vi "E725_All_VIs.vi"   [LabVIEW 2015]
doc: "This VI contains all high level and low level VIs valid for E-725. \nSee diagram for a survey of all E-725 high level and low level VIs. \nMenu / Browse / Show VI Hierarchy will show the file paths of the VIs. \nGlobal Variables are shown as Control as well as Indicator."
uses:
  Low Level/General command.llb/Controller names.ctl
  Low Level/Communication.llb/Available DLL interfaces.ctl
  Low Level/Communication.llb/Available DLLs.ctl
  Low Level/Communication.llb/Available interfaces.ctl
  Low Level/Communication.llb/Termination character.ctl
  Low Level/Analog control.llb/Available Analog Commands.ctl
  Low Level/Communication.llb/Global1.vi
  Low Level/General command.llb/Global2 (Array).vi
  Low Level/Communication.llb/Global DaisyChain.vi
  Low Level/Analog control.llb/Global Analog.vi
  Low Level/Support.llb/Unbunde/bundle interface clusters for PI Terminal.vi
panel:
  # "E-725 PI GCS LabVIEW driver set"
  # "This VI contains all high level and low level VIs valid for E-725. See diagram for a survey\nof all E-725 high level and low level VIs. Menu / Browse / Show VI Hierarchy will show\nthe file paths of the VIs. Global Variables are shown as Control as well as Indicator."
types:
  T1 = typedef "Available Analog Commands.ctl" = enum16{"INITIALIZE", "VOL?", "VOL ", "CLOSE", "MOV", "POS?", "VCO", "VCO?", "WAIT_WF", "TMN?", "TMX?", "VEL", "VEL?", "SAI?", "MVR", "ERR?", "#24", "STP", "*IDN?", "#5", "STE", "DRR?", "W_Wave", "HLP?", "W/R_Wave"}
  T2 = typedef "Termination character.ctl" = enum16{"LF", "CR", "LFCR", "CRLF"}
  T3 = typedef "Available interfaces.ctl" = u16
  T4 = typedef "Available DLLs.ctl" = u16
  T5 = typedef "Available DLL interfaces.ctl" = u16
  T6 = typedef "Controller names.ctl" = enum16{"None", "Analog", "C-702", "C-843", "C-843.PM", "C-844", "C-848", "C-865", "C-866", "C-867", "C-880", "E-516", "E-517", "E-710", "E-712", "E-725", "E-753", "E-755", "E-761", "E-816", "E-861", "F-206", "M-840", "M-850", "M-8X0", "Mercury"}
  T7 = cluster{"Conversion factor":dbl[], "Velocity":dbl[], "Velocity control mode":bool, "AO.Resolution":dbl, "Lower voltage limit (V)":dbl, "Upper voltage limit (V)":dbl, "AO_WF_T (s)":dbl, "AI Sample Rate":dbl, "AI Samples/Channel":i32, "Hyperbit":bool, "Offset (V)":dbl[], "Hyperbit StayOnPos":bool, "Gain (V)":dbl[], "Bit rate (Hz)":dbl, "PWM rate (Hz)":dbl, "HyperBit Password":string, "AO.MaxRate":dbl, "Conversion offset":dbl[]}[]
  T8 = cluster{"No. of devices":i32, "Port ID":i32, "Devices":string[], "Description":string}[]
  T9 = cluster{"Conn. axes":string[], "Controller name":T6}[]
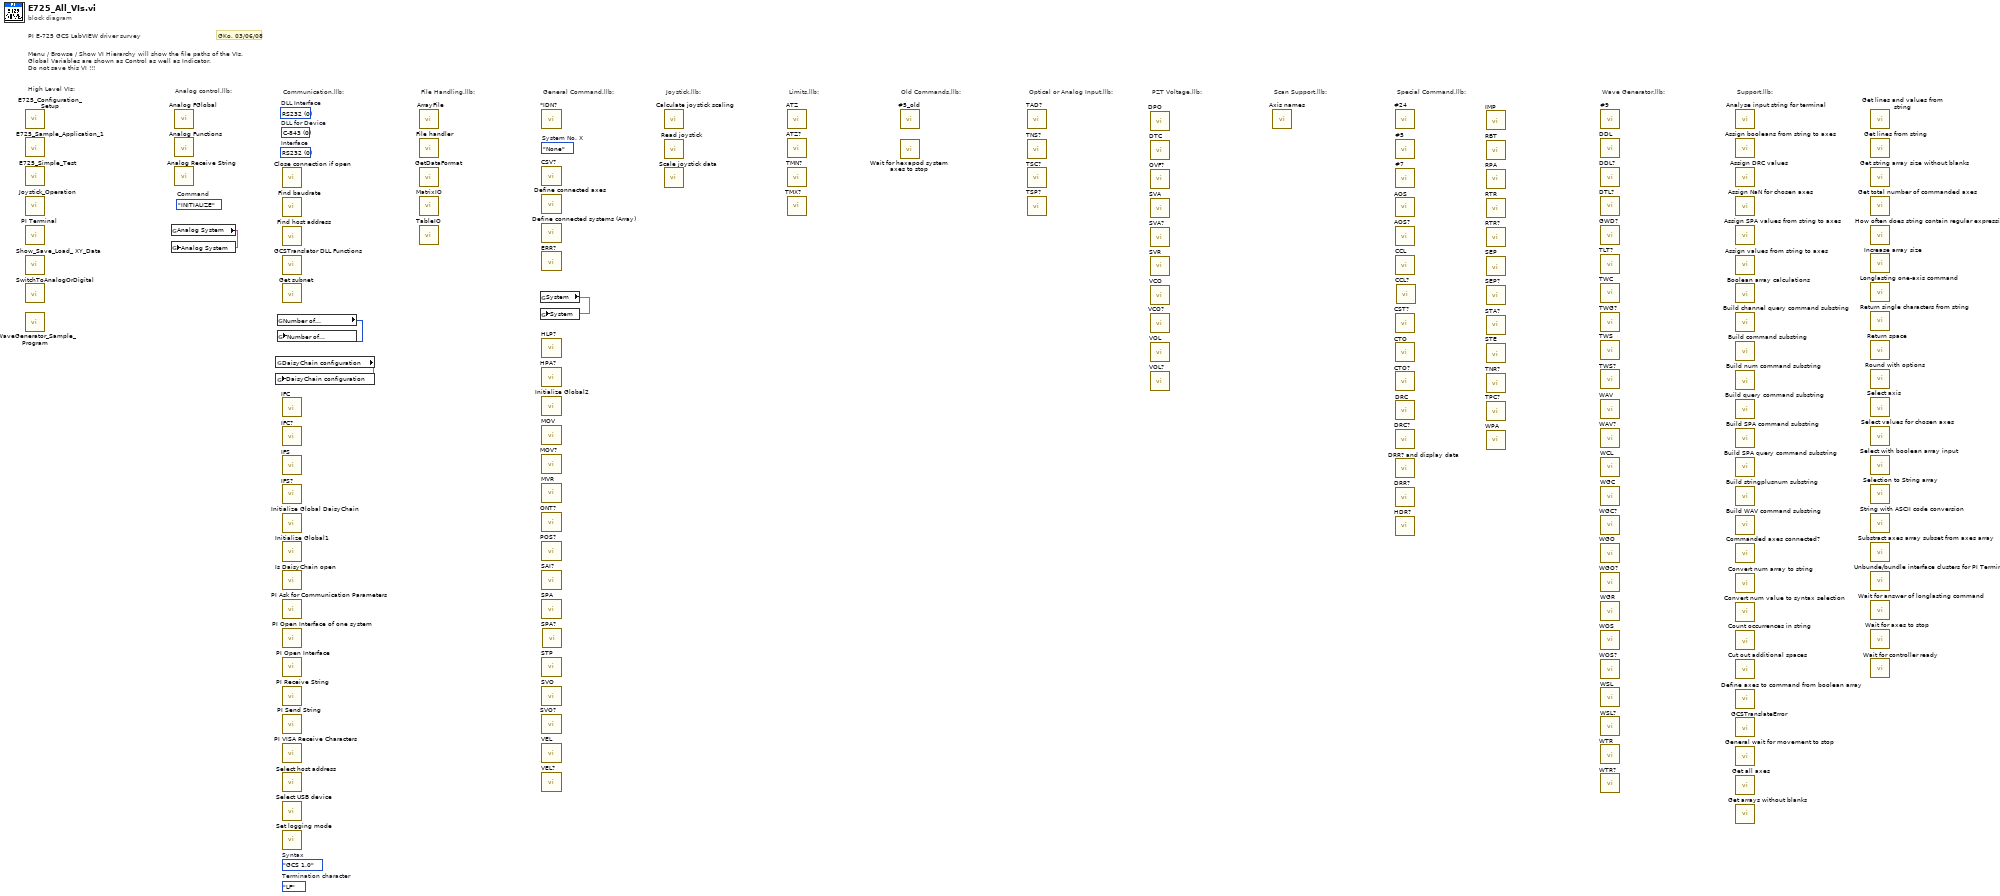
[diagram p0: block diagram]
diagram:
  (unwired) enum16{"GCS 1.0", "GCS 2.0"}."GCS 1.0"  # Syntax
  (unwired) Available_Analog_Commands."INITIALIZE"  # Command
  (unwired) Termination_character."LF"  # Termination character
  (unwired) T3 0 items=["RS232", "GPIB", "DLL", "TCP-IP"]  # Interface
  (unwired) T4 0 items=["C-843", "C-844", "E-710", "C-843.PM", "C-865", "E-761", "Mercury", "E-755", "E-753", "C-866", "E-712", "E-725", "E-861", "C-867", "E-517"]  # DLL for Device
  (unwired) T5 0 items=["RS232", "GPIB", "Board", "TCP-IP", "USB"]  # DLL Interface
  (unwired) Controller_names."None"  # System No. X
  # "GKo, 03/06/08"
  # "High Level VIs:"
  # "Analog control.llb:"
  # "Wave Generator.llb:"
  # "Support.llb:"
  # "Special Command.llb:"
  # "Scan Support.llb:"
  # "PZT Voltage.llb:"
  # "Optical or Analog Input.llb:"
  # "Old Commands.llb:"
  # "Limits.llb:"
  # "Joystick.llb:"
  # "General Command.llb:"
  # "File Handling.llb:"
  # "Menu / Browse / Show VI Hierarchy will show the file paths of the VIs. \nGlobal Variables are shown as Control as well as Indicator.\nDo not save this VI !!!"
  # "PI E-725 GCS LabVIEW driver survey"
  # "Communication.llb:"
  n1 = call "E725_Configuration_Setup.vi"() -> ()  [unwired: 15 in, 5 out]
  n2 = call "E725_Sample_Application_1.vi"() -> ()  [unwired: 1 in]
  n3 = call "E725_Simple_Test.vi"() -> ()  [unwired: 15 in, 5 out]
  n4 = call "Joystick_Operation.vi"() -> ()  [unwired: 19 in, 1 out]
  n5 = call "PI Terminal.vi"() -> ()  [unwired: 20 in]
  n6 = call "Show_Save_Load_ XY_Data.vi"() -> ()  [unwired: 19 in, 1 out]
  n7 = call "SwitchToAnalogOrDigital.vi"() -> ()  [unwired: 17 in, 3 out]
  n8 = call "WaveGenerator_Sample_Program.vi"() -> ()  [unwired: 18 in, 2 out]
  n9 = global read "Global Analog.vi" "Analog System"() -> (w1:T7)
  n10 = global write "Global Analog.vi" "Analog System"(w1) -> ()
  n11 = call "Analog FGlobal.vi"() -> ()  [unwired: 19 in, 1 out]
  n12 = call "Analog Functions.vi"() -> ()  [unwired: 17 in, 3 out]
  n13 = call "Analog Receive String.vi"() -> ()  [unwired: 18 in, 2 out]
  n14 = global read "Global DaisyChain.vi" "DaisyChain configuration"() -> (w2:T8)
  n15 = global write "Global DaisyChain.vi" "DaisyChain configuration"(w2) -> ()
  n16 = global read "Global1.vi" "Number of\nsystems"() -> (w4:i32)
  n17 = global write "Global1.vi" "Number of\nsystems"(w4) -> ()
  n18 = call "Close connection if open.vi"() -> ()  [unwired: 18 in, 2 out]
  n19 = call "Find baudrate.vi"() -> ()  [unwired: 17 in, 3 out]
  n20 = call "Find host address.vi"() -> ()  [unwired: 15 in, 5 out]
  n21 = call "GCSTranslator DLL Functions.vi"() -> ()  [unwired: 15 in, 5 out]
  n22 = call "Get subnet.vi"() -> ()  [unwired: 19 in, 1 out]
  n23 = call "IFC.vi"() -> ()  [unwired: 19 in, 1 out]
  n24 = call "IFC?.vi"() -> ()  [unwired: 18 in, 2 out]
  n25 = call "IFS.vi"() -> ()  [unwired: 19 in, 1 out]
  n26 = call "IFS?.vi"() -> ()  [unwired: 18 in, 2 out]
  n27 = call "Initialize Global DaisyChain.vi"() -> ()  [unwired: 19 in, 1 out]
  n28 = call "Initialize Global1.vi"() -> ()  [unwired: 19 in, 1 out]
  n29 = call "Is DaisyChain open.vi"() -> ()  [unwired: 17 in, 3 out]
  n30 = call "PI Ask for Communication Parameters.vi"() -> ()  [unwired: 12 in, 8 out]
  n31 = call "PI Open Interface of one system.vi"() -> ()  [unwired: 18 in, 2 out]
  n32 = call "PI Open Interface.vi"() -> ()  [unwired: 18 in, 2 out]
  n33 = call "PI Receive String.vi"() -> ()  [unwired: 17 in, 3 out]
  n34 = call "PI Send String.vi"() -> ()  [unwired: 19 in, 1 out]
  n35 = call "PI VISA Receive Characters.vi"() -> ()  [unwired: 17 in, 3 out]
  n36 = call "Select host address.vi"() -> ()  [unwired: 17 in, 3 out]
  n37 = call "Select USB device.vi"() -> ()  [unwired: 17 in, 3 out]
  n38 = call "Set logging mode.vi"() -> ()  [unwired: 19 in, 1 out]
  n39 = call "ArrayFile.vi"() -> ()  [unwired: 18 in, 2 out]
  n40 = call "File handler.vi"() -> ()  [unwired: 17 in, 3 out]
  n41 = call "GetDataFormat.vi"() -> ()  [unwired: 12 in, 8 out]
  n42 = call "MatrixIO.vi"() -> ()  [unwired: 13 in, 7 out]
  n43 = call "TableIO.vi"() -> ()  [unwired: 14 in, 6 out]
  n44 = global read "Global2 (Array).vi" "System"() -> (w3:T9)
  n45 = global write "Global2 (Array).vi" "System"(w3) -> ()
  n46 = call "*IDN?.vi"() -> ()  [unwired: 18 in, 2 out]
  n47 = call "CSV?.vi"() -> ()  [unwired: 18 in, 2 out]
  n48 = call "Define connected axes.vi"() -> ()  [unwired: 18 in, 2 out]
  n49 = call "Define connected systems (Array).vi"() -> ()  [unwired: 19 in, 1 out]
  n50 = call "ERR?.vi"() -> ()  [unwired: 18 in, 2 out]
  n51 = call "HLP?.vi"() -> ()  [unwired: 18 in, 2 out]
  n52 = call "HPA?.vi"() -> ()  [unwired: 18 in, 2 out]
  n53 = call "Initialize Global2.vi"() -> ()  [unwired: 19 in, 1 out]
  n54 = call "MOV.vi"() -> ()  [unwired: 19 in, 1 out]
  n55 = call "MOV?.vi"() -> ()  [unwired: 18 in, 2 out]
  n56 = call "MVR.vi"() -> ()  [unwired: 19 in, 1 out]
  n57 = call "ONT?.vi"() -> ()  [unwired: 18 in, 2 out]
  n58 = call "POS?.vi"() -> ()  [unwired: 18 in, 2 out]
  n59 = call "SAI?.vi"() -> ()  [unwired: 18 in, 2 out]
  n60 = call "SPA.vi"() -> ()  [unwired: 18 in, 2 out]
  n61 = call "STP.vi"() -> ()  [unwired: 19 in, 1 out]
  n62 = call "SVO.vi"() -> ()  [unwired: 19 in, 1 out]
  n63 = call "SVO?.vi"() -> ()  [unwired: 18 in, 2 out]
  n64 = call "VEL.vi"() -> ()  [unwired: 18 in, 2 out]
  n65 = call "VEL?.vi"() -> ()  [unwired: 18 in, 2 out]
  n66 = call "SPA?.vi"() -> ()  [unwired: 14 in, 6 out]
  n67 = call "Calculate joystick scaling.vi"() -> ()  [unwired: 10 in, 10 out]
  n68 = call "Read joystick.vi"() -> ()  [unwired: 15 in, 5 out]
  n69 = call "Scale joystick data.vi"() -> ()  [unwired: 18 in, 2 out]
  n70 = call "ATZ.vi"() -> ()  [unwired: 18 in, 2 out]
  n71 = call "ATZ?.vi"() -> ()  [unwired: 18 in, 2 out]
  n72 = call "TMN?.vi"() -> ()  [unwired: 18 in, 2 out]
  n73 = call "TMX?.vi"() -> ()  [unwired: 18 in, 2 out]
  n74 = call "#5_old.vi"() -> ()  [unwired: 16 in, 4 out]
  n75 = call "Wait for hexapod system axes to stop.vi"() -> ()  [unwired: 18 in, 2 out]
  n76 = call "TAD?.vi"() -> ()  [unwired: 18 in, 2 out]
  n77 = call "TNS?.vi"() -> ()  [unwired: 18 in, 2 out]
  n78 = call "TSC?.vi"() -> ()  [unwired: 18 in, 2 out]
  n79 = call "TSP?.vi"() -> ()  [unwired: 18 in, 2 out]
  n80 = call "DPO.vi"() -> ()  [unwired: 19 in, 1 out]
  n81 = call "DTC.vi"() -> ()  [unwired: 19 in, 1 out]
  n82 = call "OVF?.vi"() -> ()  [unwired: 18 in, 2 out]
  n83 = call "SVA.vi"() -> ()  [unwired: 19 in, 1 out]
  n84 = call "SVA?.vi"() -> ()  [unwired: 18 in, 2 out]
  n85 = call "SVR.vi"() -> ()  [unwired: 19 in, 1 out]
  n86 = call "VCO.vi"() -> ()  [unwired: 19 in, 1 out]
  n87 = call "VCO?.vi"() -> ()  [unwired: 18 in, 2 out]
  n88 = call "VOL.vi"() -> ()  [unwired: 19 in, 1 out]
  n89 = call "VOL?.vi"() -> ()  [unwired: 18 in, 2 out]
  n90 = call "Axis names.vi"() -> ()  [unwired: 17 in, 3 out]
  n91 = call "#24.vi"() -> ()  [unwired: 19 in, 1 out]
  n92 = call "#5.vi"() -> ()  [unwired: 18 in, 2 out]
  n93 = call "#7.vi"() -> ()  [unwired: 17 in, 3 out]
  n94 = call "AOS.vi"() -> ()  [unwired: 19 in, 1 out]
  n95 = call "AOS?.vi"() -> ()  [unwired: 18 in, 2 out]
  n96 = call "CCL.vi"() -> ()  [unwired: 18 in, 2 out]
  n97 = call "CST?.vi"() -> ()  [unwired: 18 in, 2 out]
  n98 = call "CTO.vi"() -> ()  [unwired: 18 in, 2 out]
  n99 = call "CTO?.vi"() -> ()  [unwired: 18 in, 2 out]
  n100 = call "DRC.vi"() -> ()  [unwired: 18 in, 2 out]
  n101 = call "DRC?.vi"() -> ()  [unwired: 16 in, 4 out]
  n102 = call "DRR? and display data.vi"() -> ()  [unwired: 16 in, 4 out]
  n103 = call "DRR?.vi"() -> ()  [unwired: 16 in, 4 out]
  n104 = call "HDR?.vi"() -> ()  [unwired: 18 in, 2 out]
  n105 = call "CCL?.vi"() -> ()  [unwired: 18 in, 2 out]
  n106 = call "IMP.vi"() -> ()  [unwired: 19 in, 1 out]
  n107 = call "RBT.vi"() -> ()  [unwired: 19 in, 1 out]
  n108 = call "RPA.vi"() -> ()  [unwired: 18 in, 2 out]
  n109 = call "RTR.vi"() -> ()  [unwired: 18 in, 2 out]
  n110 = call "RTR?.vi"() -> ()  [unwired: 18 in, 2 out]
  n111 = call "SEP.vi"() -> ()  [unwired: 18 in, 2 out]
  n112 = call "SEP?.vi"() -> ()  [unwired: 14 in, 6 out]
  n113 = call "STA?.vi"() -> ()  [unwired: 18 in, 2 out]
  n114 = call "STE.vi"() -> ()  [unwired: 19 in, 1 out]
  n115 = call "TNR?.vi"() -> ()  [unwired: 18 in, 2 out]
  n116 = call "TPC?.vi"() -> ()  [unwired: 18 in, 2 out]
  n117 = call "WPA.vi"() -> ()  [unwired: 18 in, 2 out]
  n118 = call "#9.vi"() -> ()  [unwired: 18 in, 2 out]
  n119 = call "DDL.vi"() -> ()  [unwired: 19 in, 1 out]
  n120 = call "DDL?.vi"() -> ()  [unwired: 18 in, 2 out]
  n121 = call "DTL?.vi"() -> ()  [unwired: 18 in, 2 out]
  n122 = call "GWD?.vi"() -> ()  [unwired: 18 in, 2 out]
  n123 = call "TLT?.vi"() -> ()  [unwired: 18 in, 2 out]
  n124 = call "TWC.vi"() -> ()  [unwired: 19 in, 1 out]
  n125 = call "TWG?.vi"() -> ()  [unwired: 18 in, 2 out]
  n126 = call "TWS.vi"() -> ()  [unwired: 18 in, 2 out]
  n127 = call "TWS?.vi"() -> ()  [unwired: 18 in, 2 out]
  n128 = call "WAV.vi"() -> ()  [unwired: 26 in, 2 out]
  n129 = call "WAV?.vi"() -> ()  [unwired: 18 in, 2 out]
  n130 = call "WCL.vi"() -> ()  [unwired: 19 in, 1 out]
  n131 = call "WGC.vi"() -> ()  [unwired: 18 in, 2 out]
  n132 = call "WGC?.vi"() -> ()  [unwired: 18 in, 2 out]
  n133 = call "WGO.vi"() -> ()  [unwired: 18 in, 2 out]
  n134 = call "WGO?.vi"() -> ()  [unwired: 18 in, 2 out]
  n135 = call "WGR.vi"() -> ()  [unwired: 19 in, 1 out]
  n136 = call "WOS.vi"() -> ()  [unwired: 19 in, 1 out]
  n137 = call "WOS?.vi"() -> ()  [unwired: 18 in, 2 out]
  n138 = call "WSL.vi"() -> ()  [unwired: 19 in, 1 out]
  n139 = call "WSL?.vi"() -> ()  [unwired: 18 in, 2 out]
  n140 = call "WTR.vi"() -> ()  [unwired: 19 in, 1 out]
  n141 = call "WTR?.vi"() -> ()  [unwired: 17 in, 3 out]
  n142 = call "Analyse input string for terminal.vi"() -> ()  [unwired: 17 in, 3 out]
  n143 = call "Assign booleans from string to axes.vi"() -> ()  [unwired: 18 in, 2 out]
  n144 = call "Assign DRC values.vi"() -> ()  [unwired: 14 in, 6 out]
  n145 = call "Assign NaN for chosen axes.vi"() -> ()  [unwired: 19 in, 1 out]
  n146 = call "Assign SPA values from string to axes.vi"() -> ()  [unwired: 14 in, 6 out]
  n147 = call "Assign values from string to axes.vi"() -> ()  [unwired: 16 in, 4 out]
  n148 = call "Boolean array calculations.vi"() -> ()  [unwired: 19 in, 1 out]
  n149 = call "Build channel query command substring.vi"() -> ()  [unwired: 16 in, 4 out]
  n150 = call "Build command substring.vi"() -> ()  [unwired: 19 in, 1 out]
  n151 = call "Build num command substring.vi"() -> ()  [unwired: 19 in, 1 out]
  n152 = call "Build query command substring.vi"() -> ()  [unwired: 17 in, 3 out]
  n153 = call "Build SPA command substring.vi"() -> ()  [unwired: 19 in, 1 out]
  n154 = call "Build SPA query command substring.vi"() -> ()  [unwired: 18 in, 2 out]
  n155 = call "Build stringplusnum substring.vi"() -> ()  [unwired: 18 in, 2 out]
  n156 = call "Build WAV command substring.vi"() -> ()  [unwired: 27 in, 1 out]
  n157 = call "Commanded axes connected?.vi"() -> ()  [unwired: 18 in, 2 out]
  n158 = call "Convert num array to string.vi"() -> ()  [unwired: 19 in, 1 out]
  n159 = call "Convert num value to syntax selection.vi"() -> ()  [unwired: 19 in, 1 out]
  n160 = call "Count occurrences in string.vi"() -> ()  [unwired: 19 in, 1 out]
  n161 = call "Cut out additional spaces.vi"() -> ()  [unwired: 19 in, 1 out]
  n162 = call "Define axes to command from boolean array.vi"() -> ()  [unwired: 17 in, 3 out]
  n163 = call "GCSTranslateError.vi"() -> ()  [unwired: 17 in, 3 out]
  n164 = call "General wait for movement to stop.vi"() -> ()  [unwired: 18 in, 2 out]
  n165 = call "Get all axes.vi"() -> ()  [unwired: 19 in, 1 out]
  n166 = call "Get arrays without blanks.vi"() -> ()  [unwired: 16 in, 4 out]
  n167 = call "Get lines and values from string.vi"() -> ()  [unwired: 17 in, 3 out]
  n168 = call "Get lines from string.vi"() -> ()  [unwired: 18 in, 2 out]
  n169 = call "Get string array size without blanks.vi"() -> ()  [unwired: 19 in, 1 out]
  n170 = call "Get total number of commanded axes.vi"() -> ()  [unwired: 16 in, 4 out]
  n171 = call "How often does string contain regular expression?.vi"() -> ()  [unwired: 19 in, 1 out]
  n172 = call "Increase array size.vi"() -> ()  [unwired: 19 in, 1 out]
  n173 = call "Longlasting one-axis command.vi"() -> ()  [unwired: 17 in, 3 out]
  n174 = call "Return single characters from string.vi"() -> ()  [unwired: 18 in, 2 out]
  n175 = call "Return space.vi"() -> ()  [unwired: 18 in, 2 out]
  n176 = call "Round with options.vi"() -> ()  [unwired: 18 in, 2 out]
  n177 = call "Select axis.vi"() -> ()  [unwired: 17 in, 3 out]
  n178 = call "Select values for chosen axes.vi"() -> ()  [unwired: 19 in, 1 out]
  n179 = call "Select with boolean array input.vi"() -> ()  [unwired: 19 in, 1 out]
  n180 = call "Selection to String array.vi"() -> ()  [unwired: 19 in, 1 out]
  n181 = call "String with ASCII code conversion.vi"() -> ()  [unwired: 19 in, 1 out]
  n182 = call "Substract axes array subset from axes array.vi"() -> ()  [unwired: 18 in, 2 out]
  n183 = call "Unbunde/bundle interface clusters for PI Terminal.vi"() -> ()  [unwired: 13 in, 7 out]
  n184 = call "Wait for answer of longlasting command.vi"() -> ()  [unwired: 17 in, 3 out]
  n185 = call "Wait for axes to stop.vi"() -> ()  [unwired: 18 in, 2 out]
  n186 = call "Wait for controller ready.vi"() -> ()  [unwired: 18 in, 2 out]
